vi "onHttpGet.vi"(6 "timeout":i32=10000, 7 "output file":path, 8 "error in":errorcluster, 10 "url":string, 11 "http-method in":refnum<class "REST Client.lvclass">) -> (0 "error out":errorcluster, 1 "body":string, 2 "headers":string, 3 "http-method out":refnum<class "REST Client.lvclass">)   [LabVIEW 2020, in "REST Client.lvlib" / "REST Client.lvclass"]
uses:
  REST Client.lvclass
  REST Client.lvclass/REST Client.ctl
  http-client/http-client.lvclass
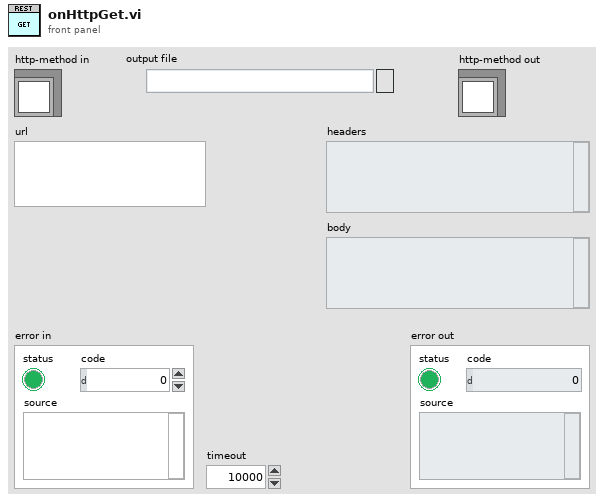
[diagram p1: front panel]
types:
  T1 = typedef "REST Client.lvlib/REST Client.lvclass/HTTP Header.ctl" = cluster{"header":T2, "value":string}
  T2 = typedef "lib_NI_Advanced HTTP Client.lvlib/Session.lvclass/Header--Combo Box.ctl" = string
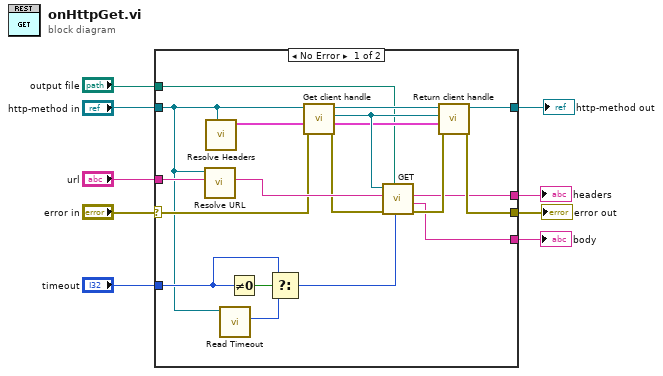
[diagram p0: block diagram]
diagram:
  n1 = case shown="No Error" "error in" {
    selector: "error in" -> [w17 w30]
    tunnel: [w13 w30] -> w6
    tunnel: [w14 w29] -> w5
    tunnel: "http-method in" -> [w16 w29]
    tunnel: "url" -> [w25 _]
    tunnel: "timeout" -> [w22 _]
    tunnel: [w12 _] -> w8
    tunnel: [w11 _] -> w7
    tunnel: "output file" -> [w10 _]
    frame No Error {
      n2 = call "Resolve URL.vi"("Path"=w25, "REST Client in"=w16) -> ("Resolved URL"=w24:string)  [unwired: 9 in]
      n3 = call "Resolve Headers.vi"("REST Client in"=w16) -> ("headers out"=w15:T1[])  [unwired: 10 in]
      n4 = call-dynamic "Read Timeout.vi"("REST Client in"=w16) -> ("Timeout"=w19:i32)  [unwired: 8 in, 2 out]
      n5 = Not Equal To 0?(x=w22) -> (x != 0?=w23:bool)
      n6 = Select(t=w22, s=w23, f=w19) -> (s? t:f=w21:i32)
      n7 = call "Get client handle.vi"("error in (no error)"=w17, "headers"=w15, "REST Client in"=w16) -> ("error out"=w20:errorcluster, "headers out"=w26:T1[], "http-client"=w27:refnum<class "http-client.lvclass">, "REST Client out"=w28:refnum<class "REST Client.lvclass">)  [unwired: 5 in]
      n8 = call "GET.vi"("timeout"=w21, "output file"=w10, "error in"=w20, "url"=w24, "http-client in"=w27) -> ("error out"=w18:errorcluster, "body"=w11:string, "headers"=w12:string)  [unwired: 2 in, 2 out]
      n9 = call "Return client handle.vi"("error in (no error)"=w18, "headers"=w26, "http-client"=w27, "REST Client in"=w28) -> ("error out"=w13:errorcluster, "REST Client out"=w14:refnum<class "REST Client.lvclass">)  [unwired: 6 in]
    }
    frame Error {
    }
  }
  "error out" <- w6
  "http-method out" <- w5
  "headers" <- w8
  "body" <- w7
